vi "Add_Pressure_Cube_Positions.vi"() -> (5 "Plug in titles":string[](array[string]), 7 "Plug in values":string[](array[string]))   [LabVIEW 2017]
uses:
  Globals/Meas_global.vi
  Globals/Trav_pos_global.vi
panel:
  out "number":i32[][](array[numeric])
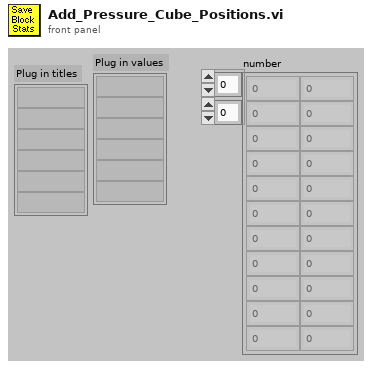
[diagram p1: front panel]
types:
  T1 = typedef "Post_Process.ctl" = enum16{"Take New Data", "Post Process Raw Data File"}
  T2 = typedef "Traverse_cluster.ctl" = cluster{"Start X":sgl, "Start Y":sgl, "Start Z":sgl, "End X":sgl, "End Y":sgl, "End Z":sgl, "No. of pts.":i32, "Spacing":T3, "Filename":path, "Tunnel Speed":dbl, "Averaging time (min)":dbl, "Extra Commands":string, "Carrier_1 Q (l/min)":dbl, "Carrier_2 Q (l/min)":dbl, "Trace Gas Concentration (%)":dbl, "Specific Arguments":string, "Comments":string, "Row No":i32, "Row Type Selector":T4, "Completion time":string, "Row Duration (mins)":dbl, "No. of Valid pts.":i32, "Meas Setup File":string}
  T3 = typedef "Spacing.ctl" = enum16{"Linear", "Log", "Gauss", "Specified", "N/A"}
  T4 = typedef "Multi_run_mode.ctl" = enum16{"Move Traverse Only", "Set Tunnel Speed Only", "Set Source Only", "Set Measurement Conditions", "Single Measurement", "Vertical Profile", "Lateral Profile", "Longitudinal Profile", "Explore Volume", "Multi-Axis Profile", "Auto Calibrate", "Meas Fast FID Bkgnd", "Check Beam Power", "Scanning Valve Measurement", "Run VI Named:", "Set ADAM Ch", "Wait (minutes)", "Send Message", "Synchronize With:", "Fall Back to this Row", "Turn Off Row Repeating", "Blank Row", "Traverse 3D Volume"}
  T5 = typedef "Analysis_info_cluster.ctl" = cluster{"Colour":u32, "Inst type":T6, "Inst name":string, "Symbol":string, "Code name":string, "Extra Info":string, "Inst Array":T7, "Extra Titles":string[], "Extra Values":string[], "U":dbl, "u^2":dbl, "u^3":dbl, "u^4":dbl, "Skew_u":dbl, "Kurt_u":dbl, "Sd Error in Mean":dbl, "% u'/U":dbl, "X":dbl, "Y":dbl, "Z":dbl, "Timescale integral Estimate":dbl, "Sd Error in Variance":dbl, "Calib File":path, "Calib Constants":dbl[], "Output Position":bool, "Full Stats":bool, "Av Sampling Rate":dbl, "Av No of Samples":dbl, "Total Meas Time (s)":dbl, "ADAM Ch Name":string, "Max value":dbl, "Min value":dbl, "Req Sample Rate Hz":dbl, "Sync Delay Time (s)":dbl, "Ch No":i16, "Device ID":string, "Use Latest Calib":bool, "Port":string, "Metadata Ch Names":string[], "Metadata Ch Values":string[]}
  T6 = typedef "Inst_type.ctl" = enum16{"Propeller anemometer", "Raw voltage", "Pressure Transducer", "Pitot-static tube", "Preston tube", "Hot wire", "Cross wire 1", "Cross wire 2", "Generic Linear", "Generic Polynomial", "Generic BackPoly", "Fast FID", "Thermocouple", "Cold wire", "Pulsed Wire", "LDA Vel", "LDA Tran time", "LDA Arr time", "Microphone"}
  T7 = typedef "Instrument_Array.ctl" = enum16{"PWA", "LDA", "Analogue"}
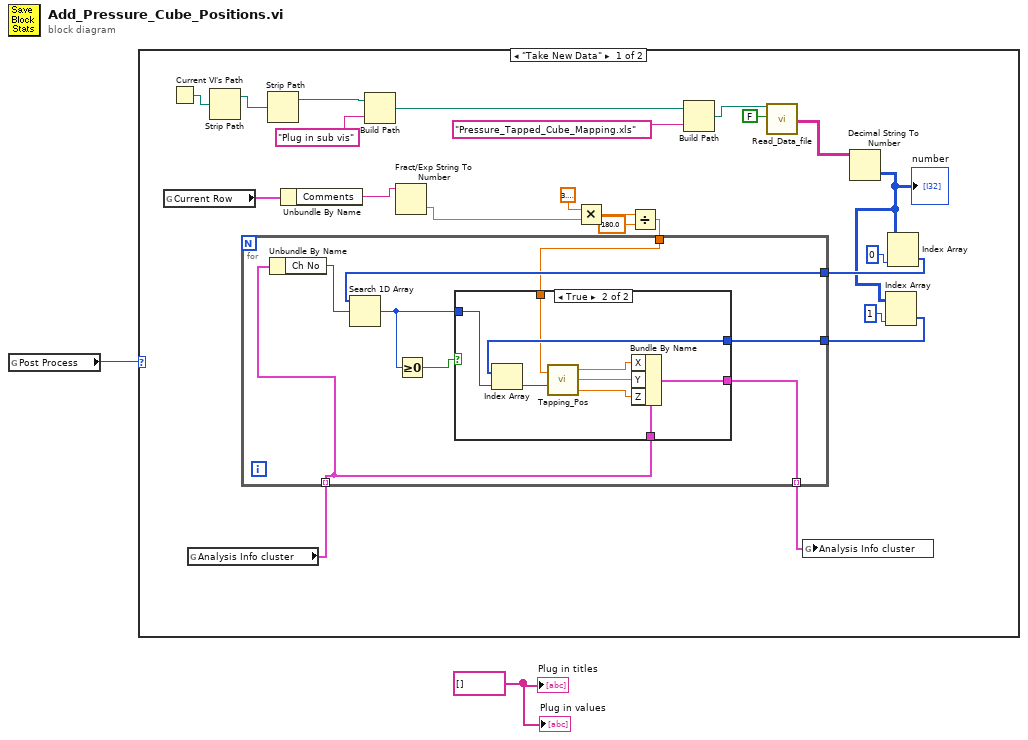
[diagram p0: block diagram]
diagram:
  w2 = string[] [] ("Plug in titles")
  n1 = global read "Meas_global.vi" "Post Process"() -> (w1:T1)
  n2 = case shown="\"Take New Data\"" w1 {
    frame "Take New Data" {
      n3 = global read "Trav_pos_global.vi" "Current Row"() -> (w5:T2)
      n4 = Current VI's Path() -> (path=w23:path)
      n5 = global read "Meas_global.vi" "Analysis Info cluster"() -> (w25:T5[])
      n6 = Strip Path(path=w23) -> (stripped path=w22:path)  [unwired: 1 out]
      n7 = Strip Path(path=w22) -> (stripped path=w21:path)  [unwired: 1 out]
      n8 = Unbundle By Name(w5) -> ("Comments"=w4:string)
      n9 = Build Path(base path=w21, name or relative path="Plug in sub vis") -> (appended path=w19:path)
      n10 = Fract/Exp String To Number(string=w4) -> (number=w3:dbl)  [unwired: 3 in, 1 out]
      n11 = Multiply(x=3.141592653589793, y=w3) -> (x*y=w9:dbl)
      n12 = Divide(x=w9, y=180.0) -> (x/y=w7:dbl)
      n13 = Build Path(base path=w19, name or relative path="Pressure_Tapped_Cube_Mapping.xls") -> (appended path=w17:path)
      n14 = call "Read_Data_file.vi"("Results file"=w17, "Delete First Rows?"=FALSE) -> ("Channel Values Out"=w16:string[][])  [unwired: 7 in, 10 out]
      n15 = Decimal String To Number(string=w16) -> (number=w12:i32[][])  [unwired: 2 in, 1 out]
      "number" <- w12
      n16 = Index Array(array=w12, index (col)=1 ("index (row)")) -> (element=w11:i32[])  [unwired: 1 in]
      n17 = Index Array(array=w12, index (col)=0 ("index (row)")) -> (element=w15:i32[])  [unwired: 1 in]
      n18 = for {
        tunnel: w25 -> [w26] mode=indexing
        tunnel: [w33] -> w24 mode=indexing
        tunnel: w15 -> [w32]
        tunnel: w11 -> [w30]
        tunnel: w7 -> [w27]
        n19 = Unbundle By Name(w26) -> ("Ch No"=w31:i16)
        n20 = Search 1D Array(1D array=w32, element=w31) -> (index of element=w29:i32)  [unwired: 1 in]
        n21 = Greater Or Equal To 0?(x=w29) -> (x >= 0?=w28:bool)
        n22 = case shown="True" w28 {
          tunnel: w26 -> [w34 w43]
          tunnel: [w34 w42] -> w33
          tunnel: w30 -> [_ w38]
          tunnel: w29 -> [_ w36]
          tunnel: w27 -> [_ w35]
          frame False {
          }
          frame True {
            n23 = Index Array(array=w38, index=w36) -> (element=w37:i32)
            n24 = call "Tapping_Pos.vi"("Orientation (radians)"=w35, "Tapping Number"=w37) -> ("X"=w39:sgl, "Y"=w40:sgl, "Z"=w41:sgl)
            n25 = Bundle By Name(cluster=w43, "X"=w39, "Y"=w40, "Z"=w41) -> (w42:T5)
          }
        }
      }
      n26 = global write "Meas_global.vi" "Analysis Info cluster"(w24) -> ()
    }
    frame "Post Process Raw Data File" {
    }
  }
  "Plug in values" <- w2
  "Plug in titles" <- w2
